vi "Validate Fixed Header.vi"(8 "error in (no error)":errorcluster, 11 "PUBLISH in":refnum<class "PUBLISH.lvclass">) -> (0 "error out":errorcluster, 1 "Valid":bool, 3 "PUBLISH out":refnum<class "PUBLISH.lvclass">)   [LabVIEW 2013, in "MQTT_Control_Packets.lvlib" / "PUBLISH.lvclass"]
uses:
  PUBLISH.lvclass
  ControlPacket/ControlPacket.lvclass/ControlPacket.ctl
  ControlPacket/ControlPacket.lvclass
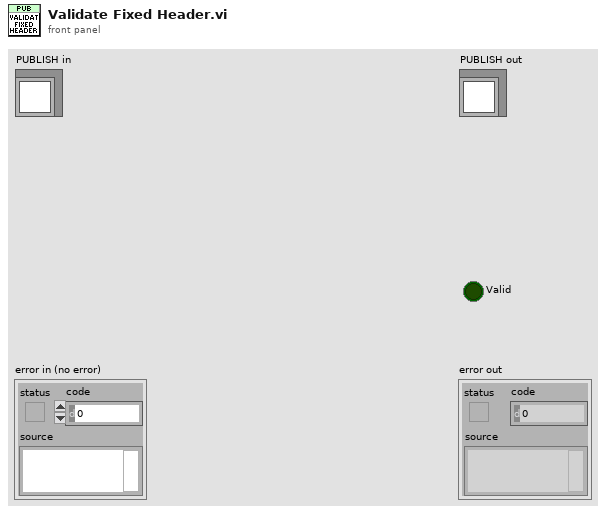
[diagram p1: front panel]
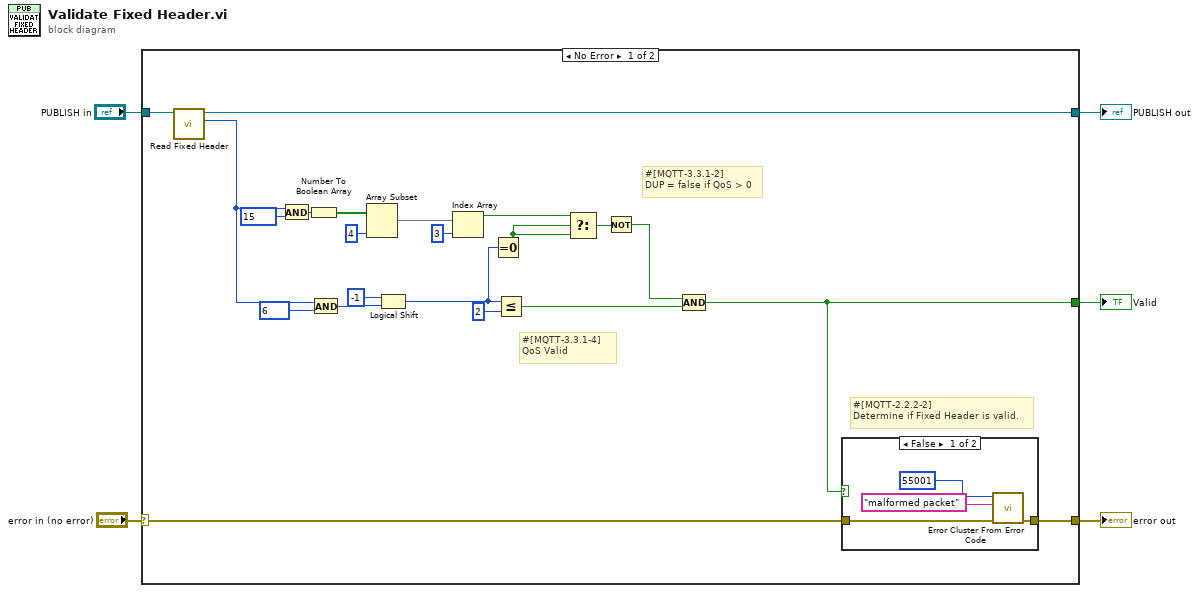
[diagram p0: block diagram]
diagram:
  n1 = case shown="No Error" "error in (no error)" {
    selector: "error in (no error)" -> [w8 w34]
    tunnel: [w7 w34] -> w5
    tunnel: [w6 _] -> w4
    tunnel: [w10 w33] -> w3
    tunnel: "PUBLISH in" -> [w9 w33]
    frame No Error {
      # "#[MQTT-2.2.2-2]\nDetermine if Fixed Header is valid."
      # "#[MQTT-3.3.1-2]\nDUP = false if QoS > 0"
      # "#[MQTT-3.3.1-4]\nQoS Valid"
      n2 = call "Read Fixed Header.vi"("ControlPacket in"=w9) -> ("Fixed Header"=w11:u8, "ControlPacket out"=w10:refnum<class "PUBLISH.lvclass">)  [unwired: 9 in]
      n3 = And(x=w11, y=u8 15) -> (x .and. y?=w26:u8)
      n4 = Number To Boolean Array(number=w26) -> (Boolean array=w24:bool[])
      n5 = And(x=w11, y=u8 6) -> (x .and. y?=w21:u8)
      n6 = Array Subset(array=w24, length=4) -> (w17:bool[])  [unwired: 1 in]
      n7 = Logical Shift(y=i16 -1, x=w21) -> (x << y=w18:u8)
      n8 = Index Array(array=w17, index=3) -> (element=w15:bool)
      n9 = Equal To 0?(x=w18) -> (x = 0?=w14:bool)
      n10 = Less Or Equal?(x=w18, y=u8 2) -> (x <= y?=w19:bool)
      n11 = Select(t=w15, s=w14, f=w14) -> (s? t:f=w13:bool)
      n12 = Not(x=w13) -> (.not. x?=w12:bool)
      n13 = Compound Arithmetic op=AND(w12, w19) -> (w6:bool)
      n14 = case shown="False" w6 {
        tunnel: [w29 w32] -> w7
        tunnel: w8 -> [w28 w32]
        frame False {
          n15 = call <vilib>:"Error Cluster From Error Code.vi"("error in (no error)"=w28, "error message (\"\")"="malformed packet" ("error message (\"\")"), "error code (0)"=55001) -> ("error out"=w29:errorcluster)  [unwired: 6 in]
        }
        frame True {
        }
      }
    }
    frame Error {
    }
  }
  "Valid" <- w4
  "error out" <- w5
  "PUBLISH out" <- w3
